vi "BRig_RT__Case_Idle__State_UploadSettings_checkFile.vi"(11 "input_dataName":string="dataExp") -> (1 "output_Iexist":bool, 2 "output_dataPath":path)   [LabVIEW 2014]
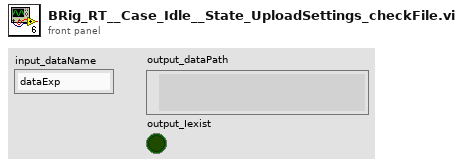
[diagram p1: front panel]
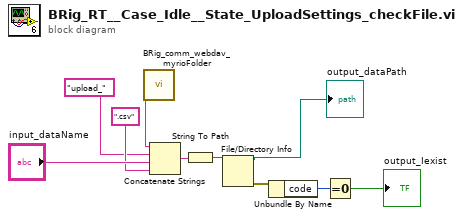
[diagram p0: block diagram]
diagram:
  n1 = call "BRig_comm_webdav_myrioFolder.vi"() -> ("output_myrioFolder"=w8:string)  [unwired: 11 in]
  n2 = Concatenate Strings(w8, "upload_" ("string"), "input_dataName", ".csv" ("string")) -> (w6:string)
  n3 = String To Path(string=w6) -> (path=w5:path)
  n4 = File/Directory Info(path=w5) -> (path out=→"output_dataPath":path, error out=w3:errorcluster)  [unwired: 1 in, 5 out]
  n5 = Unbundle By Name(w3) -> ("code"=w2:i32)
  n6 = Equal To 0?(x=w2) -> (x = 0?=→"output_Iexist":bool)
